vi "ziModGetScopeWave.vi"(8 "Error In":errorcluster, 10 "ModResults":T3, 11 "ModHandle In":T6 {"ModHandle" format="0x%08x"; "Conn" format="0x%08x"}) -> (0 "Error Out":errorcluster, 1 "ModScopeWaveGrid":T1[][](array[typedef]) {"dt (s)" format="%#_6p"}, 2 "ModScopeWave":T2[][](array[typedef]) {"dt (s)" format="%#_6p"}, 3 "ModHandle Out":T6 {"ModHandle" format="0x%08x"; "Conn" format="0x%08x"})   [LabVIEW 2018, in "Zurich Instruments LabOne.lvlib"]
doc: "Use this vi to get IntegerData from a ModResult returned from ziModGetNextNode.vi. It return an array of IntegerData."
uses:
  Zurich Instruments LabOne.lvlib
  Data/ziTypeIntegerDataTS.ctl
  <instrlib>/Zurich Instruments LabOne/Private/ziLV64.framework
  Data/ziTypeScopeWave.ctl
  Data/ziTypeScopeWaveGrid.ctl
  ziTypeModHandle.ctl
  Data/ziTypePollType.ctl
  ziTypeModResults.ctl
  ziTypeModGenericHeader.ctl
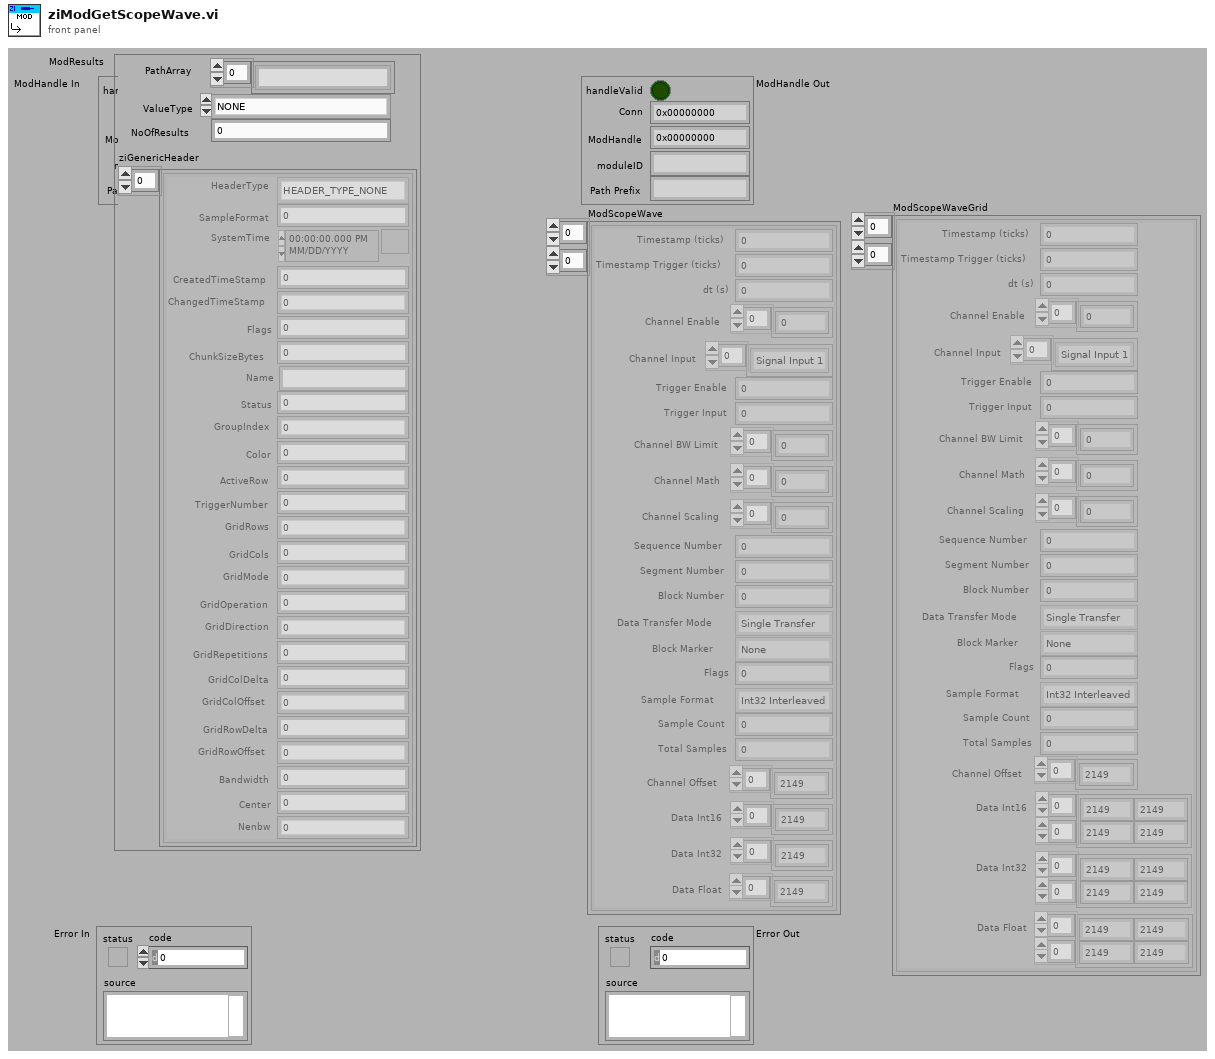
[diagram p1: front panel]
types:
  T1 = typedef "Zurich Instruments LabOne.lvlib/ziTypeScopeWaveGrid.ctl" = cluster{"Timestamp (ticks)":u64, "Timestamp Trigger (ticks)":u64, "dt (s)":dbl, "Channel Enable":u8[], "Channel Input":enum8{"Signal Input 1", "Signal Input 2", "Trigger Input 1", "Trigger Input 2", "Aux Output 1", "Aux Output 2", "Aux Output 3", "Aux Output 4", "Aux Input 1", "Aux Input 2"}[], "Trigger Enable":u64, "Trigger Input":u64, "Channel BW Limit":u8[], "Channel Math":u8[], "Channel Scaling":sgl[], "Sequence Number":u32, "Segment Number":u32, "Block Number":u32, "Data Transfer Mode":enum8{"Single Transfer", "Block Transfer", "Continuous Transfer", "FFT Single Transfer"}, "Block Marker":enum8{"None", "End of Block"}, "Flags":u8, "Sample Format":enum8{"Int16", "Int32", "Float32", "reserved", "Int16 Interleaved", "Int32 Interleaved", "Float32 Interleaved"}, "Sample Count":u32, "Channel Offset":dbl[], "Data Int16":i16[][], "Data Int32":i32[][], "Data Float":sgl[][], "Total Samples":u32}
  T2 = typedef "Zurich Instruments LabOne.lvlib/ziTypeScopeWave.ctl" = cluster{"Timestamp (ticks)":u64, "Timestamp Trigger (ticks)":u64, "dt (s)":dbl, "Channel Enable":u8[], "Channel Input":enum8{"Signal Input 1", "Signal Input 2", "Trigger Input 1", "Trigger Input 2", "Aux Output 1", "Aux Output 2", "Aux Output 3", "Aux Output 4", "Aux Input 1", "Aux Input 2"}[], "Trigger Enable":u64, "Trigger Input":u64, "Channel BW Limit":u8[], "Channel Math":u8[], "Channel Scaling":sgl[], "Sequence Number":u32, "Segment Number":u32, "Block Number":u32, "Data Transfer Mode":enum8{"Single Transfer", "Block Transfer", "Continuous Transfer", "FFT Single Transfer"}, "Block Marker":enum8{"None", "End of Block"}, "Flags":u8, "Sample Format":enum8{"Int16", "Int32", "Float32", "reserved", "Int16 Interleaved", "Int32 Interleaved", "Float32 Interleaved"}, "Sample Count":u32, "Channel Offset":dbl[], "Data Int16":i16[], "Data Int32":i32[], "Data Float":sgl[], "Total Samples":u64}
  T3 = typedef "Zurich Instruments LabOne.lvlib/ziTypeModResults.ctl" = cluster{"PathArray":string[], "ValueType":T4, "NoOfResults":u64, "ziGenericHeader":T5[]}
  T4 = typedef "Zurich Instruments LabOne.lvlib/ziTypePollType.ctl" = enum16{"NONE", "DOUBLE_DATA", "INTEGER_DATA", "DEMOD_SAMPLE", "SCOPE_WAVE_HF2", "AUXIN_SAMPLE", "DIO_SAMPLE", "BYTE_ARRAY", "PWA_WAVE", "9", "10", "11", "12", "13", "14", "15", "TREE_CHANGE_DEPRI", "17", "ERROR", "19", "20", "21", "22", "23", "24", "25", "26", "27", "28", "29", "30", "31", "DOUBLE_DATA_TS", "INTEGER_DATA_TS", "34", "SCOPE_WAVE", "SCOPE_WAVE_EX", "37", "BYTE_ARRAY_TS", "39", "40", "41", "42", "43", "44", "45", "CNT_DATA", "47", "TREE_CHANGE", "49", "50", "51", "52", "53", "54", "55", "56", "57", "58", "59", "60", "61", "62", "63", "SWEEPER_DATA", "SPECTRUM_DATA", "ADVISOR_DATA", "VECTOR_DATA", "IMP_DATA"}
  T5 = typedef "Zurich Instruments LabOne.lvlib/ziTypeModGenericHeader.ctl" = cluster{"HeaderType":enum8{"HEADER_TYPE_NONE", "HEADER_TYPE_SWTRIGGER", "HEADER_TYPE_SWEEPER"}, "SampleFormat":u8, "SystemTime":timestamp, "CreatedTimeStamp":u64, "ChangedTimeStamp":u64, "Flags":u32, "ChunkSizeBytes":u64, "Name":string, "Status":u32, "GroupIndex":u32, "Color":u32, "ActiveRow":u32, "TriggerNumber":u64, "GridRows":u32, "GridCols":u32, "GridMode":u32, "GridOperation":u32, "GridDirection":u32, "GridRepetitions":u32, "GridColDelta":dbl, "GridColOffset":dbl, "GridRowDelta":dbl, "GridRowOffset":dbl, "Bandwidth":dbl, "Center":dbl, "Nenbw":dbl}
  T6 = typedef "Zurich Instruments LabOne.lvlib/ziTypeModHandle.ctl" = cluster{"handleValid":bool, "Conn":u64, "ModHandle":u64, "moduleID":string, "Path Prefix":string}
  T7 = enum8{"Signal Input 1", "Signal Input 2", "Trigger Input 1", "Trigger Input 2", "Aux Output 1", "Aux Output 2", "Aux Output 3", "Aux Output 4", "Aux Input 1", "Aux Input 2"}[]
  T8 = enum8{"Single Transfer", "Block Transfer", "Continuous Transfer", "FFT Single Transfer"}
  T9 = enum8{"Int16", "Int32", "Float32", "reserved", "Int16 Interleaved", "Int32 Interleaved", "Float32 Interleaved"}
  T10 = typedef "Zurich Instruments LabOne.lvlib/ziTypeIntegerDataTS.ctl" = cluster{"Timestamp (ticks)":u64[], "Value":i64[]}
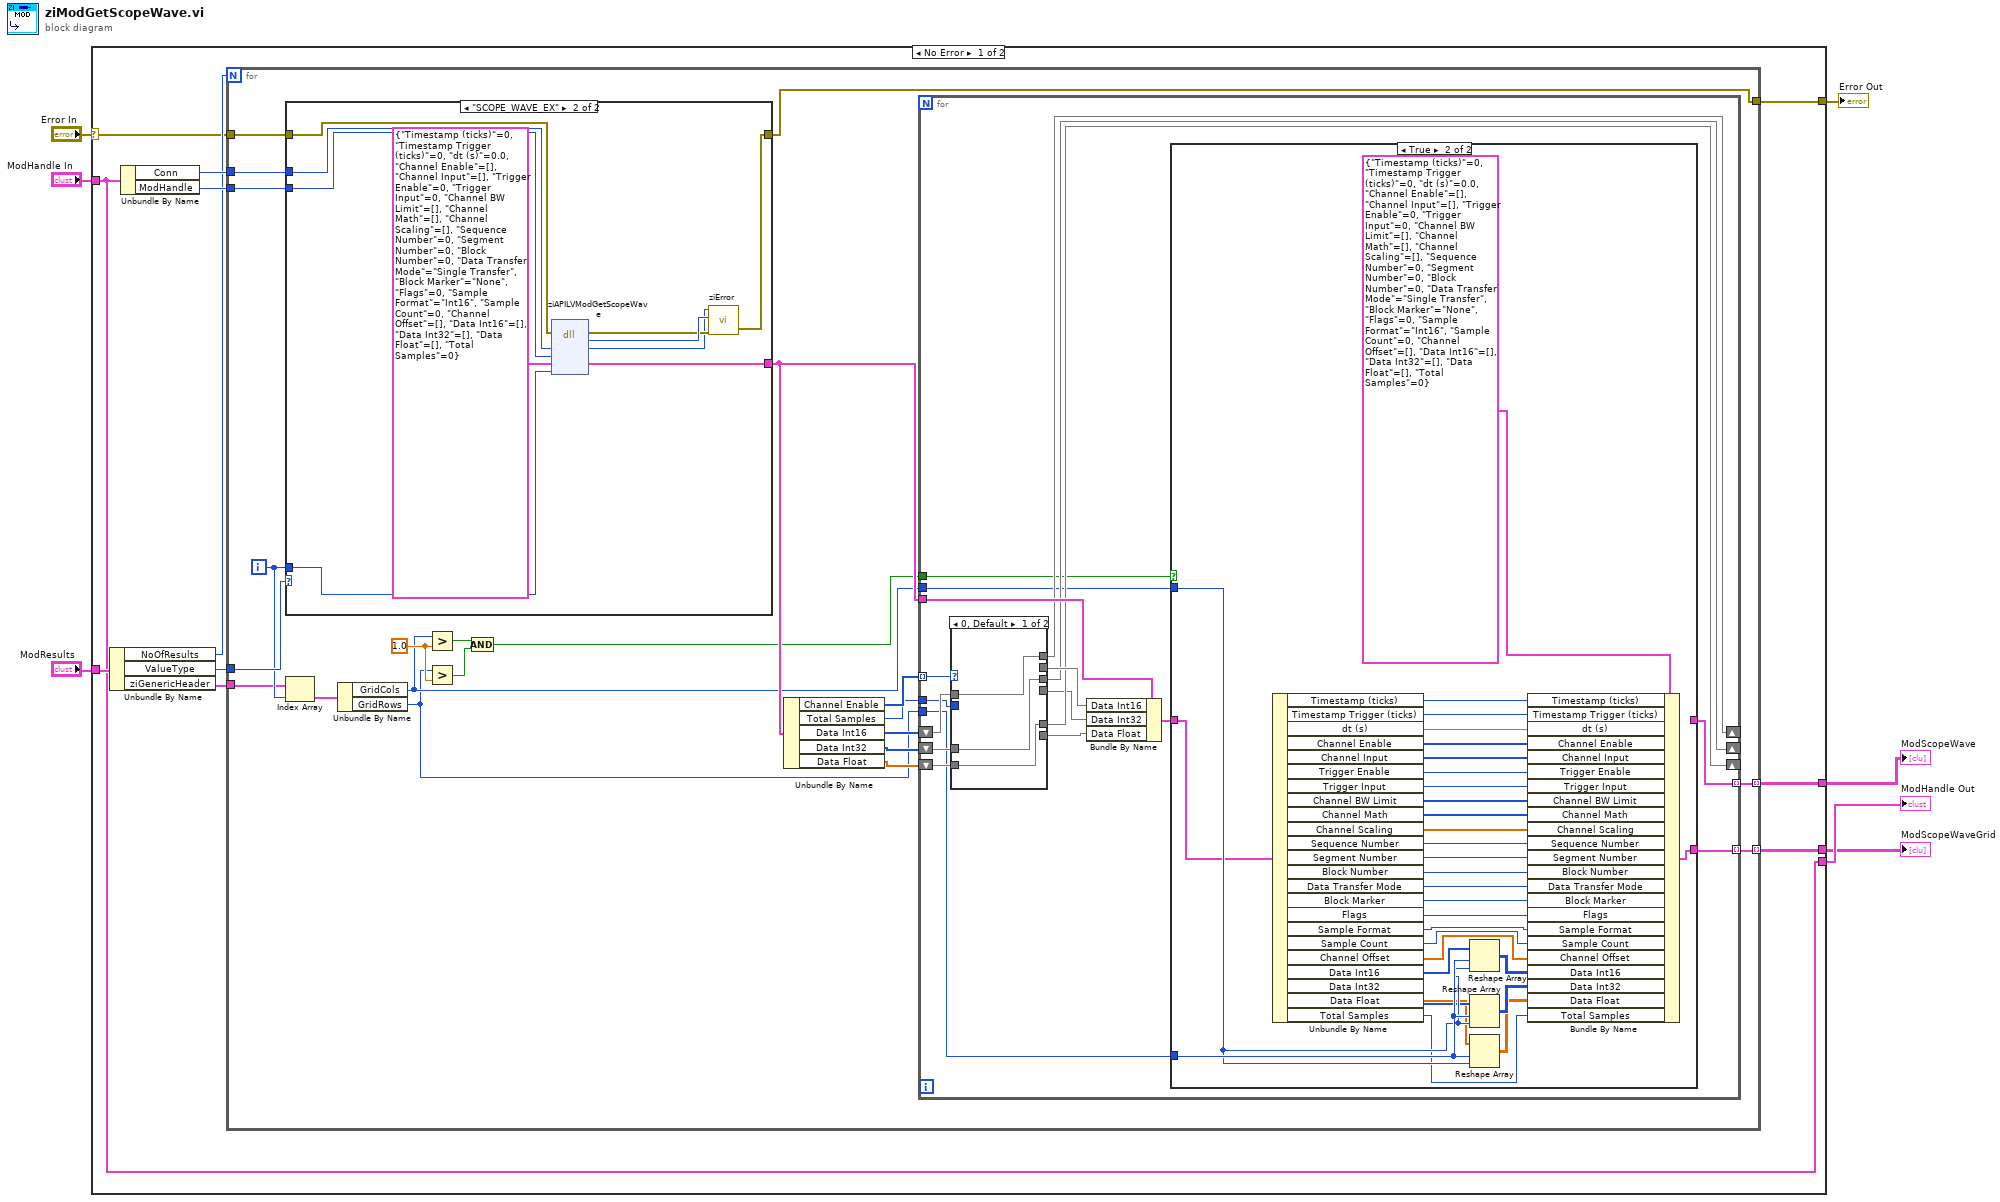
[diagram p0: block diagram]
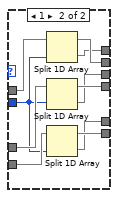
[diagram p3: hidden frame]
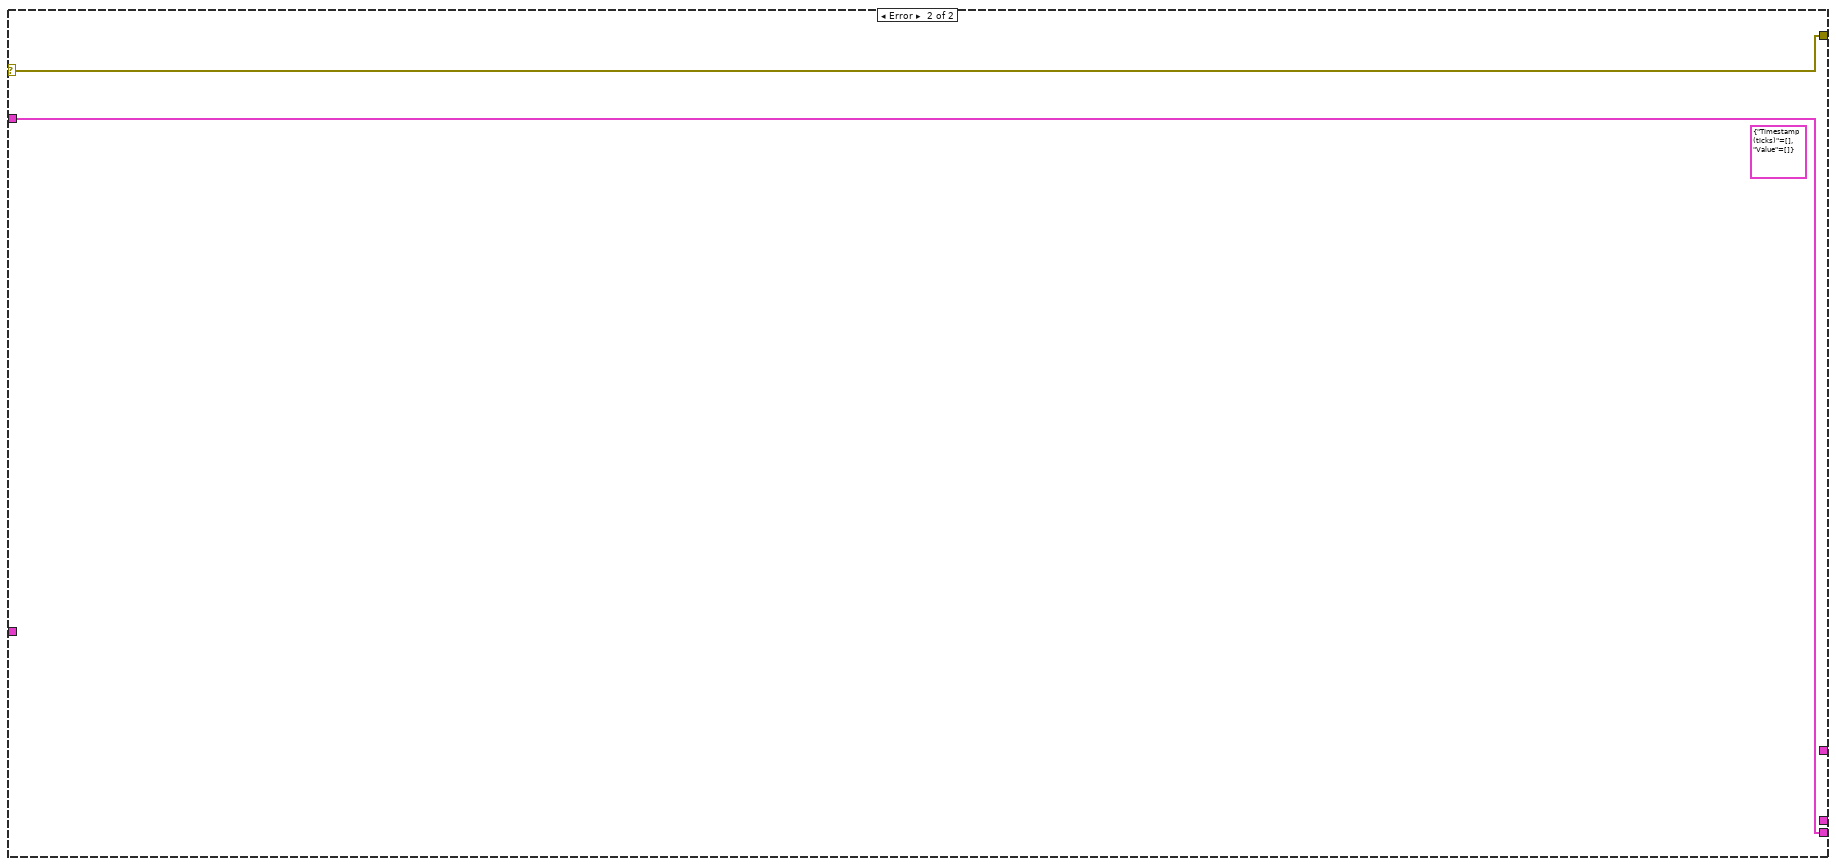
[diagram p5: hidden frame]
diagram:
  n1 = case shown="No Error" "Error In" {
    selector: "Error In" -> [w13 w115]
    tunnel: [w14 w115] -> w3
    tunnel: [w12 w116] -> w6
    tunnel: "ModHandle In" -> [w12 w116]
    tunnel: "ModResults" -> [w16 _]
    tunnel: [w9 _] -> w2
    tunnel: [w8 _] -> w1
    frame No Error {
      n2 = Unbundle By Name(w16) -> ("NoOfResults"=w15:u64, "ValueType"=w11:T4, "ziGenericHeader"=w10:T5[])
      n3 = Unbundle By Name(w12) -> ("Conn"=w18:u64, "ModHandle"=w17:u64)
      n4 = for {
        N: w15 -> [_]
        tunnel: w18 -> [w40]
        tunnel: w17 -> [w39]
        tunnel: [w38] -> w14
        tunnel: w13 -> [w37]
        tunnel: w11 -> [w36]
        tunnel: w10 -> [w30]
        tunnel: [w28] -> w9 mode=indexing
        tunnel: [w19] -> w8 mode=indexing
        i -> [w31]
        w35 = 1.0 ("y")
        n5 = case shown="\"SCOPE_WAVE_EX\"" w36 {
          tunnel: w40 -> [_ w114]
          tunnel: w39 -> [_ w113]
          tunnel: w31 -> [_ w112]
          tunnel: [w104 w111] -> w38
          tunnel: w37 -> [w104 w108]
          tunnel: [_ w105] -> w29
          frame "NONE", Default {
          }
          frame "SCOPE_WAVE_EX" {
            n6 = dll-call lib="Applications/National Instruments/LabVIEW 2019 64-bit/instr.lib/Zurich Instruments LabOne/Private/ziLV*.*" fn="ziAPILVModGetScopeWave"(error in=w108, "Conn"=w114, "ModHandle"=w113, "ScopeWave"=T2 {"Timestamp (ticks)"=0, "Timestamp Trigger (ticks)"=0, "dt (s)"=0.0, "Channel Enable"=[], "Channel Input"=[], "Trigger Enable"=0, "Trigger Input"=0, "Channel BW Limit"=[], "Channel Math"=[], "Channel Scaling"=[], "Sequence Number"=0, "Segment Number"=0, "Block Number"=0, "Data Transfer Mode"=enum."Single Transfer", "Block Marker"=enum."None", "Flags"=0, "Sample Format"=enum."Int16", "Sample Count"=0, "Channel Offset"=[], "Data Int16"=[], "Data Int32"=[], "Data Float"=[], "Total Samples"=0}, "chunk_idx"=w112) -> (error out=w109:errorcluster, "return type"=w110:u32, "Conn"=w107:u64, "ScopeWave"=w105:T2)  [unwired: 4 in, 1 out]
            n7 = call "ziError.vi"("Conn"=w107, "ziErrorCode"=w110, "Error In"=w109) -> ("Error Out"=w111:errorcluster)  [unwired: 2 in, 1 out]
          }
        }
        n8 = Index Array(array=w30, index=w31) -> (element=w32:T5)
        n9 = Unbundle By Name(w32) -> ("GridCols"=w21:u32, "GridRows"=w20:u32)
        n10 = Greater?(x=w21, y=w35) -> (0:w33:bool)
        n11 = Greater?(x=w20, y=w35) -> (0:w34:bool)
        n12 = And(x=w33, y=w34) -> (x .and. y?=w22:bool)
        n13 = Unbundle By Name(w29) -> ("Channel Enable"=w27:u8[], "Total Samples"=w26:u64, "Data Int16"=w25:i16[], "Data Int32"=w24:i32[], "Data Float"=w23:sgl[])
        n14 = for {
          tunnel: w29 -> [w58]
          tunnel: [w41] -> w28 mode=indexing
          tunnel: w26 -> [w47]
          shift-right: [w56] -> _
          shift-left: w25 -> [w57]
          tunnel: w27 -> [w55] mode=indexing
          shift-right: [w50] -> _
          shift-left: w23 -> [w52]
          shift-right: [w51] -> _
          shift-left: w24 -> [w53]
          tunnel: w22 -> [w46]
          tunnel: w21 -> [w45]
          tunnel: w20 -> [w44]
          tunnel: [w43] -> w19 mode=indexing
          n15 = case shown="0, Default" w55 {
            tunnel: w57 -> [w93 w103]
            tunnel: w47 -> [_ w100]
            tunnel: [w93 w94] -> w56
            tunnel: [_ w95] -> w54
            tunnel: w53 -> [w91 w102]
            tunnel: w52 -> [w92 w101]
            tunnel: [w91 w96] -> w51
            tunnel: [w92 w98] -> w50
            tunnel: [_ w97] -> w49
            tunnel: [_ w99] -> w48
            frame 0, Default {
            }
            frame 1 {
              n16 = Split 1D Array(array=w103, index=w100) -> (first subarray=w95:i16[], second subarray=w94:i16[])
              n17 = Split 1D Array(array=w102, index=w100) -> (first subarray=w97:i32[], second subarray=w96:i32[])
              n18 = Split 1D Array(array=w101, index=w100) -> (first subarray=w99:sgl[], second subarray=w98:sgl[])
            }
          }
          n19 = Bundle By Name(cluster=w58, "Data Int16"=w54, "Data Int32"=w49, "Data Float"=w48) -> (w42:T2)
          n20 = case shown="True" w46 {
            tunnel: w44 -> [_ w88]
            tunnel: w45 -> [_ w87]
            tunnel: [_ w90] -> w43
            tunnel: w42 -> [w59 w80]
            tunnel: [w59 _] -> w41
            frame False {
            }
            frame True {
              n21 = Unbundle By Name(w80) -> ("Timestamp (ticks)"=w79:u64, "Timestamp Trigger (ticks)"=w78:u64, "dt (s)"=w77:dbl, "Channel Enable"=w76:u8[], "Channel Input"=w75:T7, "Trigger Enable"=w74:u64, "Trigger Input"=w73:u64, "Channel BW Limit"=w72:u8[], "Channel Math"=w71:u8[], "Channel Scaling"=w70:sgl[], "Sequence Number"=w69:u32, "Segment Number"=w68:u32, "Block Number"=w67:u32, "Data Transfer Mode"=w66:T8, "Block Marker"=w65:enum8{"None", "End of Block"}, "Flags"=w64:u8, "Sample Format"=w63:T9, "Sample Count"=w62:u32, "Channel Offset"=w61:dbl[], "Data Int16"=w86:i16[], "Data Int32"=w85:i32[], "Data Float"=w84:sgl[], "Total Samples"=w60:u64)
              n22 = Reshape Array(w86, w88, w87) -> (w83:i16[][])
              n23 = Reshape Array(w85, w88, w87) -> (w82:i32[][])
              n24 = Reshape Array(w84, w88, w87) -> (w81:sgl[][])
              n25 = Bundle By Name(cluster=T1 {"Timestamp (ticks)"=0, "Timestamp Trigger (ticks)"=0, "dt (s)"=0.0, "Channel Enable"=[], "Channel Input"=[], "Trigger Enable"=0, "Trigger Input"=0, "Channel BW Limit"=[], "Channel Math"=[], "Channel Scaling"=[], "Sequence Number"=0, "Segment Number"=0, "Block Number"=0, "Data Transfer Mode"=enum."Single Transfer", "Block Marker"=enum."None", "Flags"=0, "Sample Format"=enum."Int16", "Sample Count"=0, "Channel Offset"=[], "Data Int16"=[], "Data Int32"=[], "Data Float"=[], "Total Samples"=0} ("IntegerData"), "Timestamp (ticks)"=w79, "Timestamp Trigger (ticks)"=w78, "dt (s)"=w77, "Channel Enable"=w76, "Channel Input"=w75, "Trigger Enable"=w74, "Trigger Input"=w73, "Channel BW Limit"=w72, "Channel Math"=w71, "Channel Scaling"=w70, "Sequence Number"=w69, "Segment Number"=w68, "Block Number"=w67, "Data Transfer Mode"=w66, "Block Marker"=w65, "Flags"=w64, "Sample Format"=w63, "Sample Count"=w62, "Channel Offset"=w61, "Data Int16"=w83, "Data Int32"=w82, "Data Float"=w81, "Total Samples"=w60) -> (w90:T1)
            }
          }
        }
      }
    }
    frame Error {
      (unwired) T10 {"Timestamp (ticks)"=[], "Value"=[]} ("IntegerSample 2")
    }
  }
  "Error Out" <- w3
  "ModHandle Out" <- w6
  "ModScopeWave" <- w2
  "ModScopeWaveGrid" <- w1
